vi "PQ Example SELECT Clusters.vi"() -> ()   [LabVIEW 2016]
uses:
  Connection/PQ Connection.lvclass
  Result/PQ Result.lvclass
  Connection/Execute Command (Result).vi
panel:
  out "Array":T1(array[cluster])
  in  "Connection Strings":string="host=localhost port=5433 dbname=mydb user=postgres password=******"
  out "error out":errorcluster
  # "Run \"PQ Example Many INSERTs.vi\" first to generate data to SELECT from"
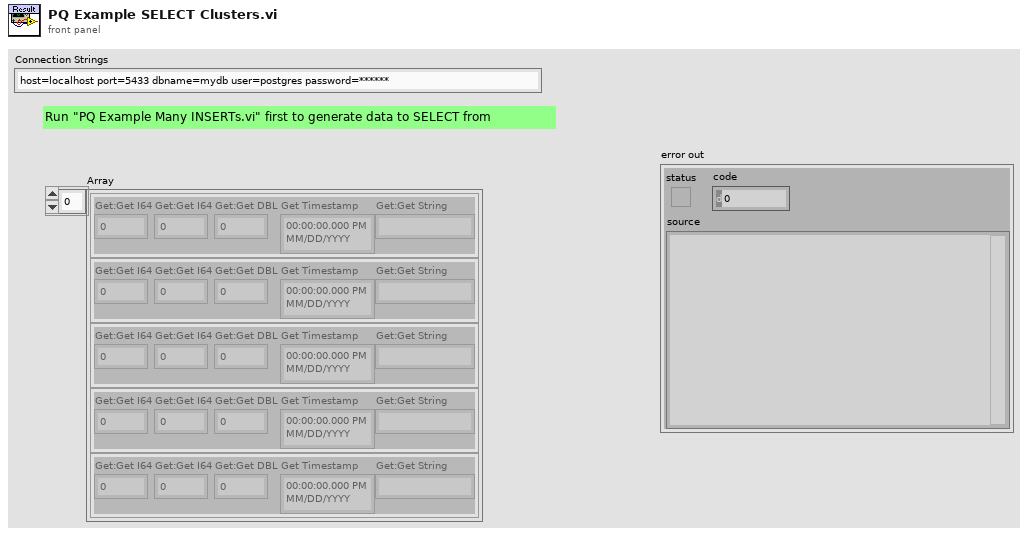
[diagram p1: front panel]
types:
  T1 = cluster{"Get:Get I64":i64, "Get:Get I64":i64, "Get:Get DBL":dbl, "Get Timestamp":timestamp, "Get:Get String":string}[]
  T2 = cluster{"Get:Get I64":i64, "Get:Get I64":i64, "Get:Get DBL":dbl, "Get:Get Timestamp":timestamp, "Get:Get String":string}
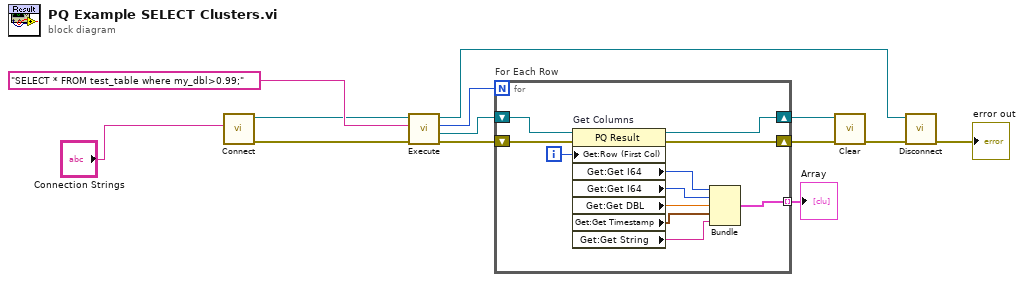
[diagram p0: block diagram]
diagram:
  n1 = call "Connect.vi"("Connection Strings"="Connection Strings") -> ("error out"=w8:errorcluster, "PQ Connection out"=w10:refnum<class "PQ Connection.lvclass">)  [unwired: 9 in]
  n2 = call-poly "Execute.vi"("error in (no error)"=w8, "SQL"="SELECT * FROM test_table where my_dbl>0.99;" ("command"), "PQ Connection in"=w10) -> ("error out"=w3:errorcluster, "First Result with Rows returned"=w5:refnum<class "PQ Result.lvclass">, "Number of Rows"=w4:i32, "PQ Connection out"=w9:refnum<class "PQ Connection.lvclass">)  [unwired: 5 in]
  n3 = for "For Each Row" {
    N: w4 -> [_]
    shift-right: [w24] -> w6
    shift-left: w5 -> [w17]
    shift-right: [w23] -> w2
    shift-left: w3 -> [w16]
    tunnel: [w18] -> w1 mode=indexing
    i -> [w15]
    n4 = property on="Get Columns" class="PQ Result"(reference=w17, error in=w16, "Get:Row (First Col)"=w15) -> (reference out=w24:refnum<class "PQ Result.lvclass">, error out=w23:errorcluster, "Get:Get I64"=w22:i64, "Get:Get I64"=w21:i64, "Get:Get DBL"=w20:dbl, "Get:Get Timestamp"=w19:timestamp, "Get:Get String"=w14:string)
    n5 = Bundle("Get:Get I64"=w22, "Get:Get I64"=w21, "Get:Get DBL"=w20, "Get:Get Timestamp"=w19, "Get:Get String"=w14) -> (w18:T2)  [unwired: 1 in]
  }
  "Array" <- w1
  n6 = call "Clear.vi"("error in (no error)"=w2, "PQ Result  in"=w6) -> ("error out"=w11:errorcluster)  [unwired: 9 in]
  n7 = call-dynamic "Disconnect.vi"("error in (no error)"=w11, "PQ Connection in"=w9) -> ("error out"=→"error out":errorcluster)  [unwired: 9 in]
